vi "GetFileVersion_Win.vi"(8 "error in (no error)":errorcluster, 11 "Exe Path":path) -> (0 "error out":errorcluster, 2 "File Info Out":T1, 3 "Exe Path Out":path)   [LabVIEW 2020]
doc: "This VI can obtain information about an existing executable, such as its version, product name, and so on, or it can be called as a subVI from a VI that will be built into an executable to obtain information about that executable.\n\nTo obtain version information about an existing executable, enter a path to an executable into Exe Path and run the Vi.\n\nCall this VI as a subVI from a VI that you will build into an executable and leave the path input unwired to obtain the version information about the built executable."
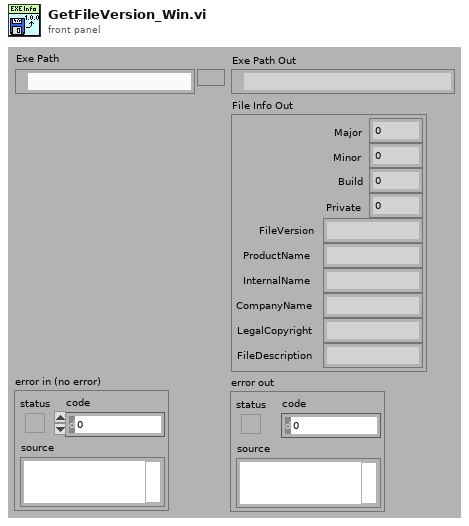
[diagram p1: front panel]
types:
  T1 = cluster{"Major":i32, "Minor":i32, "Build":i32, "Private":i32, "FileVersion":string, "ProductName":string, "InternalName":string, "CompanyName":string, "LegalCopyright":string, "FileDescription":string}
  T2 = typedef "FileVersionInformation.ctl" = cluster{"FileVersion":string, "ProductName":string, "InternalName":string, "CompanyName":string, "LegalCopyright":string, "FileDescription":string}
  T3 = cluster{i32, i32, i32, i32, "FileVersion":string, "ProductName":string, "InternalName":string, "CompanyName":string, "LegalCopyright":string, "FileDescription":string}
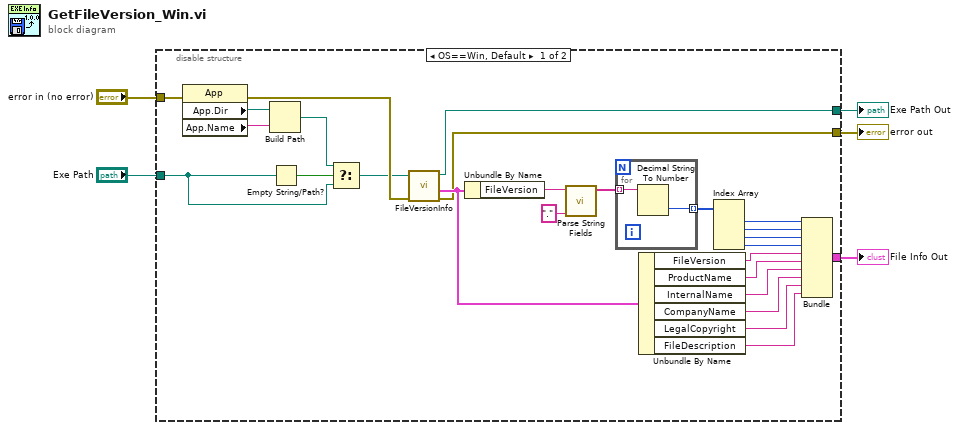
[diagram p0: block diagram]
diagram:
  n1 = disable-structure shown="OS==Win, Default" {
    disable-tunnel: "Exe Path" -> [w28 w34]
    disable-tunnel: "error in (no error)" -> [w26 w35]
    disable-tunnel: [w24 w34] -> w3
    disable-tunnel: [w7 _] -> w2
    disable-tunnel: [w6 w35] -> w1
    frame condition #0 (active) {
      n2 = property class="App"(error in=w26) -> (error out=w25:errorcluster, "App.Dir"=w31:path, "App.Name"=w30:string)  [unwired: 1 in, 1 out]
      n3 = Build Path(base path=w31, name or relative path=w30) -> (appended path=w27:path)
      n4 = Empty String/Path?(string/path=w28) -> (empty?=w29:bool)
      n5 = Select(t=w27, s=w29, f=w28) -> (s? t:f=w23:path)
      n6 = call <vilib>:"FileVersionInfo.vi"("error in (no error)"=w25, "Application Path in"=w23) -> ("error out"=w6:errorcluster, "FileVersionInfo Out"=w14:T2, "Application Path out"=w24:path)  [unwired: 6 in, 1 out]
      n7 = Unbundle By Name(w14) -> ("FileVersion"=w22:string)
      n8 = call "Parse String Fields.vi"("Separator"=".", "String"=w22) -> ("Fields"=w20:string[])  [unwired: 8 in, 1 out]
      n9 = for {
        tunnel: w20 -> [w33] mode=indexing
        tunnel: [w32] -> w19 mode=indexing
        n10 = Decimal String To Number(string=w33) -> (number=w32:i32)  [unwired: 2 in, 1 out]
      }
      n11 = Unbundle By Name(w14) -> ("FileVersion"=w12:string, "ProductName"=w13:string, "InternalName"=w11:string, "CompanyName"=w10:string, "LegalCopyright"=w9:string, "FileDescription"=w8:string)
      n12 = Index Array(array=w19) -> (element #1=w18:i32, element #2=w17:i32, element #3=w16:i32, element #4=w15:i32)  [unwired: 4 in]
      n13 = Bundle(w18, w17, w16, w15, "FileVersion"=w12, "ProductName"=w13, "InternalName"=w11, "CompanyName"=w10, "LegalCopyright"=w9, "FileDescription"=w8) -> (w7:T3)  [unwired: 1 in]
    }
    frame condition #1 {
    }
  }
  "error out" <- w1
  "Exe Path Out" <- w3
  "File Info Out" <- w2
